vi "Get Computer Name.vi"(8 "error in (no error)":errorcluster) -> (0 "error out":errorcluster, 2 "name":string)   [LabVIEW 2019, in "Control Experiment.lvclass"]
uses:
  Control Experiment.lvclass
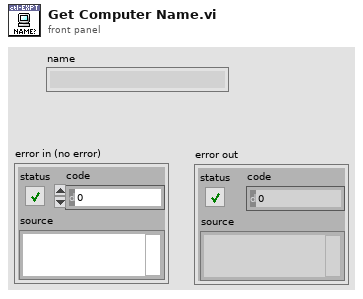
[diagram p1: front panel]
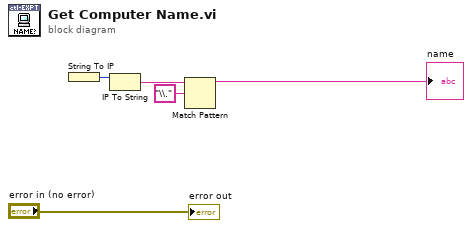
[diagram p0: block diagram]
diagram:
  n1 = String To IP() -> (0:w2:u32)  [unwired: 1 in]
  n2 = IP To String(2:w2) -> (0:w3:string)  [unwired: 1 in]
  n3 = Match Pattern(string=w3, regular expression="\\.") -> (before substring=→"name":string)  [unwired: 1 in, 3 out]
  "error out" <- "error in (no error)"
